vi "Basic Math.vi"() -> ()   [LabVIEW 2018]
doc: "Shows how to send numerical arrays to Python, and perform basic mathematical operations on them."
panel:
  out "Result":dbl
  in  "stop":bool
  in  "Input B":dbl(knob) scale=0.0..10.0
  in  "Input A":dbl(knob) scale=0.0..10.0
  out "Waveform Chart":dbl(graph)
  out "error out":errorcluster
  # "Basic Math & Using Arrays"
  # "This example shows how to get started using numerical arrays with\nthe Toolkit.  LabVIEW types are automatically converted to \"NumPy\"\narrays, which are the standard numerical type in the Python world.\n\nWe take an array of numbers, and then call a Python function which\nsquares them.\n\nTry changing the number representation for \"Data In\" or\n\"Squared Result\" to integer, or changing the Unpack.vi drop-down\nselection to \"Int Array\", and see what happens.\n\nThis VI pops up the Python console by default, so you can see some\nhelpful information printed by the function, including the type\nof the array received by Python."
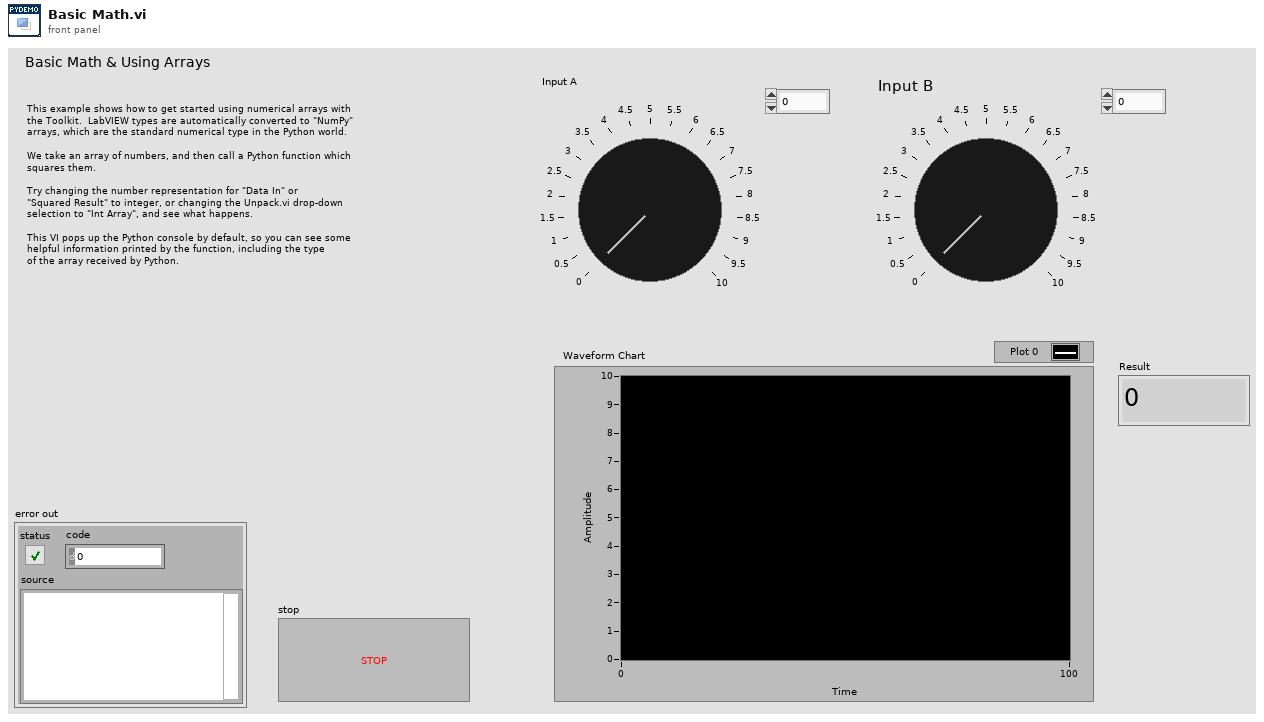
[diagram p1: front panel]
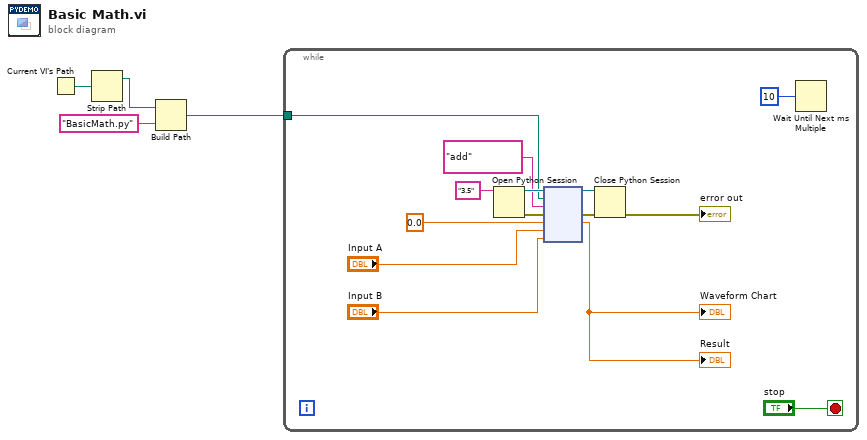
[diagram p0: block diagram]
diagram:
  n1 = Current VI's Path() -> (path=w4:path)
  n2 = Strip Path(path=w4) -> (stripped path=w3:path)  [unwired: 1 out]
  n3 = Build Path(base path=w3, name or relative path="BasicMath.py") -> (appended path=w1:path)
  n4 = while {
    tunnel: w1 -> [w12]
    stop <- "stop" stop-if-true
    n5 = Open Python Session(python version="3.5" ("Python version")) -> (session out=w17:refnum<k35>, error out=w14:errorcluster)  [unwired: 2 in]
    n6 = node(w17, w12, "add" ("Function or Method Name"), w14, 0.0, "Input A", "Input B") -> (w15:refnum<k35>, w13:errorcluster, →"Waveform Chart" →"Result":dbl)  [unwired: 2 in, 2 out]
    n7 = Close Python Session(session in=w15, error in=w13) -> (11:→"error out":errorcluster)
    n8 = Wait Until Next ms Multiple(millisecond multiple=u32 10) -> ()  [unwired: 1 out]
  }
